vi "ChangeChanCurveRefGain.vi"(8 "错误输入（无错误）":errorcluster, 10 "曲线参考点增益":u16, 11 "曲线参考点索引":u8) -> (0 "错误输出":errorcluster)   [LabVIEW 2014]
uses:
  X86Dll/ZXUTConfigMgr.dll
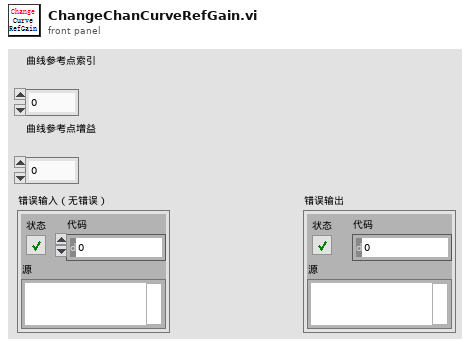
[diagram p1: front panel]
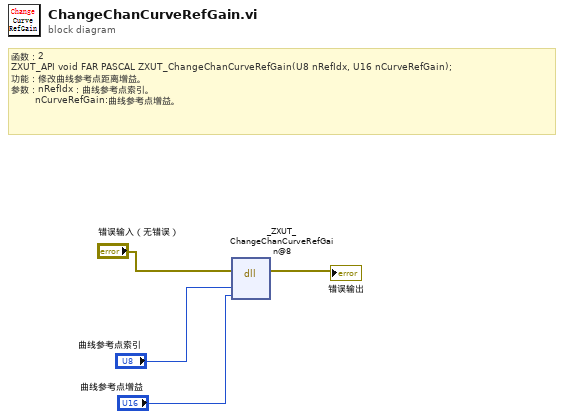
[diagram p0: block diagram]
diagram:
  # "函数：2\nZXUT_API void\tFAR PASCAL ZXUT_ChangeChanCurveRefGain(U8 nRefIdx, U16 nCurveRefGain);\n功能：修改曲线参考点距离增益。\n参数：nRefIdx：曲线参考点索引。\n        nCurveRefGain:曲线参考点增益。"
  n1 = dll-call lib="D:/Software/Utrasonic on-line monitoring/X86Dll/ZXUTConfigMgr.dll" fn="_ZXUT_ChangeChanCurveRefGain@8"(error in="错误输入（无错误）", "nRefIdx"="曲线参考点索引", "nCurveRefGain"="曲线参考点增益") -> (error out=→"错误输出":errorcluster)  [unwired: 5 in, 1 out]
